vi "Read Spec Data.vi"(0 "section":string, 5 "key":string, 9 "default value":dbl format="%#_13g", 11 "error in (no error)":errorcluster) -> (4 "value":dbl, 15 "error out":errorcluster)   [LabVIEW 2024, in "devicePowerSequencerCoreLogic.lvlib"]
uses:
  devicePowerSequencerCoreLogic.lvlib
  <vilib>/Utility/config.llb/Read Key (Double).vi
  <vilib>/Utility/config.llb/NI_LVConfig.lvlib
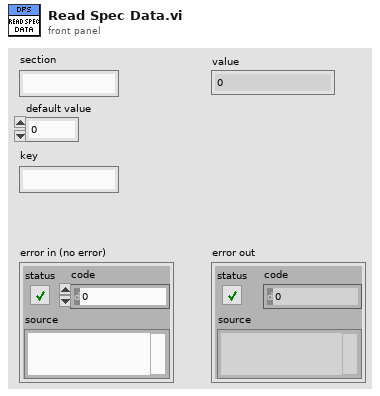
[diagram p1: front panel]
types:
  T1 = typedef "NI_LVConfig.lvlib/Config Data RefNum.ctl" = refnum<k1>
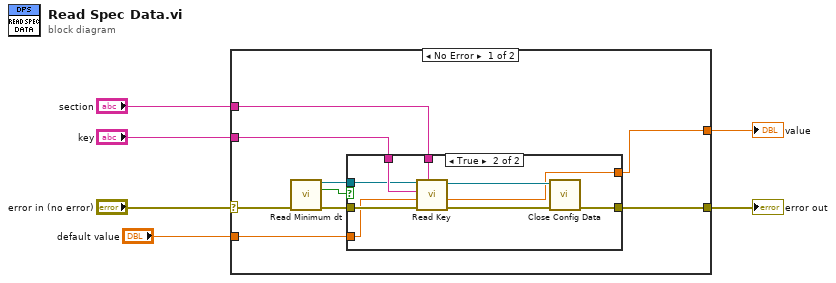
[diagram p0: block diagram]
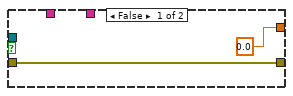
[diagram p2: hidden frame]
diagram:
  n1 = case shown="No Error" "error in (no error)" {
    selector: "error in (no error)" -> [w10 w27]
    tunnel: "section" -> [w15 _]
    tunnel: "key" -> [w14 _]
    tunnel: [w13 _] -> w3
    tunnel: [w12 w27] -> w2
    tunnel: "default value" -> [w7 _]
    frame No Error {
      n2 = call "Read Minimum dt.vi"("error in (no error)"=w10) -> ("refnum"=w11:T1, "File Exist?"=w8:bool, "error out"=w9:errorcluster)  [unwired: 12 in]
      n3 = case shown="True" w8 {
        tunnel: w15 -> [_ w24]
        tunnel: w14 -> [_ w23]
        tunnel: [0.0 ("value") w22] -> w13
        tunnel: [w16 w21] -> w12
        tunnel: w11 -> [_ w20]
        tunnel: w9 -> [w16 w19]
        tunnel: w7 -> [_ w18]
        frame False {
        }
        frame True {
          n4 = call-poly <vilib>:"Read Key.vi"("section"=w24, "error in (no error)"=w19, "default value"=w18, "key"=w23, "refnum"=w20) -> ("error out"=w26:errorcluster, "value"=w22:dbl, "refnum out"=w25:T1)  [unwired: 3 in, 1 out]
          n5 = call <vilib>:"Close Config Data.vi"("error in (no error)"=w26, "refnum"=w25) -> ("error out"=w21:errorcluster)  [unwired: 8 in, 1 out]
        }
      }
    }
    frame Error {
    }
  }
  "error out" <- w2
  "value" <- w3
